vi "Convert Variant to string.vi"(10 "variant":variant) -> (2 "data string":string)   [LabVIEW 2015]
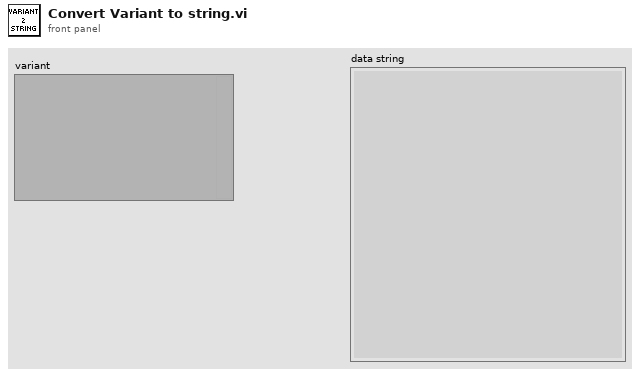
[diagram p1: front panel]
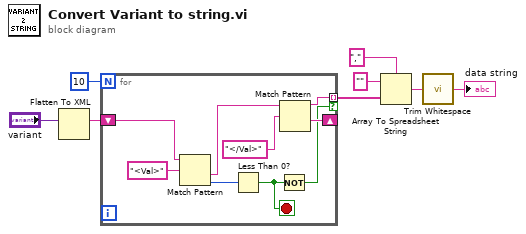
[diagram p0: block diagram]
diagram:
  n1 = Flatten To XML(anything="variant") -> (xml string=w8:string)
  n2 = for {
    N: 10 -> [_]
    shift-right: [w11] -> _
    shift-left: w8 -> [w14]
    tunnel: [w12] -> w5 mode=indexing if=w9
    stop <- w10 stop-if-true
    n3 = Match Pattern(string=w14, regular expression="<Val>") -> (after substring=w15:string, offset past match=w13:i32)  [unwired: 1 in, 2 out]
    n4 = Less Than 0?(x=w13) -> (x < 0?=w10:bool)
    n5 = Not(x=w10) -> (.not. x?=w9:bool)
    n6 = Match Pattern(string=w15, regular expression="</Val>") -> (before substring=w12:string, after substring=w11:string)  [unwired: 1 in, 2 out]
  }
  n7 = Array To Spreadsheet String(delimiter (Tab)=",", array=w5, 3:"" ("format string")) -> (spreadsheet string=w4:string)
  n8 = call <vilib>:"Trim Whitespace.vi"("string"=w4) -> ("trimmed string"=→"data string":string)  [unwired: 1 in]
